vi "Update Servo Parameters.vi"(8 "error in":errorcluster, 11 "tCRD in":refnum<class "Aircraft OPCCRD.lvclass">) -> (0 "error out":errorcluster, 3 "tCRD out":refnum<class "Aircraft OPCCRD.lvclass">)   [LabVIEW 2015, in "Aircraft OPCCRD.lvclass"]
uses:
  Aircraft OPCCRD.lvclass
  Switch/Servo Switch.lvclass
  Reusable/Switch/Switch.lvclass
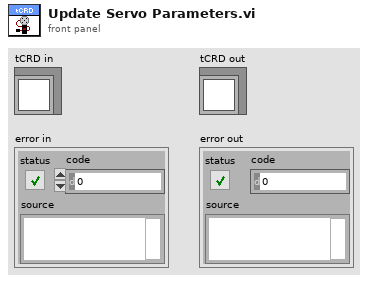
[diagram p1: front panel]
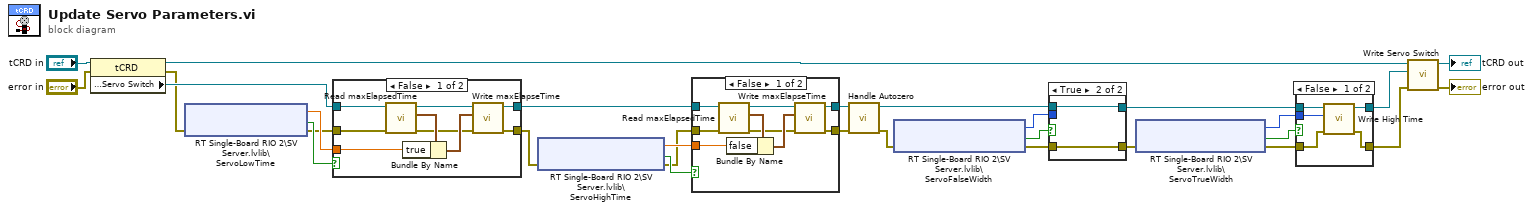
[diagram p0: block diagram]
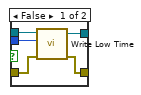
[diagram p3: hidden frame]
diagram:
  n1 = property class="tCRD"(reference="tCRD in", error in="error in") -> (reference out=w4:refnum<class "Aircraft OPCCRD.lvclass">, error out=w1:errorcluster, "Accessors:Servo Switch"=w3:refnum<class "Servo Switch.lvclass">)
  n2 = shared-variable "RT Single-Board RIO 2\\SV Server.lvlib\\ServoLowTime"(error in=w1) -> (w17:sgl, error out=w11:errorcluster, w16:bool)  [unwired: 1 in]
  n3 = case shown="False" w16 {
    tunnel: w11 -> [w34 w40]
    tunnel: [w31 w39] -> w18
    tunnel: w17 -> [w30 _]
    tunnel: w3 -> [w38 w39]
    tunnel: [w32 w40] -> w10
    frame False {
      n4 = call "Read maxElapsedTime.vi"("error in"=w34, "Switch in"=w38) -> ("error out"=w33:errorcluster, "maxElapsedTime"=w37:cluster{"true":sgl, "false":sgl}, "Switch out"=w36:refnum<class "Servo Switch.lvclass">)  [unwired: 7 in]
      n5 = Bundle By Name(cluster=w37, "true"=w30) -> (w35:cluster{"true":sgl, "false":sgl})
      n6 = call "Write maxElapseTime.vi"("error in"=w33, "maxElapsedTime"=w35, "Switch in"=w36) -> ("error out"=w32:errorcluster, "Switch out"=w31:refnum<class "Servo Switch.lvclass">)  [unwired: 7 in]
    }
    frame True {
    }
  }
  n7 = shared-variable "RT Single-Board RIO 2\\SV Server.lvlib\\ServoHighTime"(error in=w10) -> (w19:sgl, error out=w9:errorcluster, w20:bool)  [unwired: 1 in]
  n8 = case shown="False" w20 {
    tunnel: w18 -> [w48 w51]
    tunnel: [w44 w51] -> w21
    tunnel: w19 -> [w49 _]
    tunnel: w9 -> [w47 w50]
    tunnel: [w41 w50] -> w8
    frame False {
      n9 = call "Read maxElapsedTime.vi"("error in"=w47, "Switch in"=w48) -> ("error out"=w42:errorcluster, "maxElapsedTime"=w46:cluster{"true":sgl, "false":sgl}, "Switch out"=w43:refnum<class "Servo Switch.lvclass">)  [unwired: 7 in]
      n10 = Bundle By Name(cluster=w46, "false"=w49) -> (w45:cluster{"true":sgl, "false":sgl})
      n11 = call "Write maxElapseTime.vi"("error in"=w42, "maxElapsedTime"=w45, "Switch in"=w43) -> ("error out"=w41:errorcluster, "Switch out"=w44:refnum<class "Servo Switch.lvclass">)  [unwired: 7 in]
    }
    frame True {
    }
  }
  n12 = call "Handle Autozero.vi"("error in"=w8, "Servo Switch in"=w21) -> ("error out"=w28:errorcluster, "Servo Switch out"=w27:refnum<class "Servo Switch.lvclass">)  [unwired: 8 in]
  n13 = shared-variable "RT Single-Board RIO 2\\SV Server.lvlib\\ServoFalseWidth"(error in=w28) -> (w23:u32, error out=w29:errorcluster, w22:bool)  [unwired: 1 in]
  n14 = case shown="True" w22 {
    tunnel: w27 -> [w56 w58]
    tunnel: w23 -> [w55 _]
    tunnel: [w54 w58] -> w24
    tunnel: w29 -> [w53 w57]
    tunnel: [w52 w57] -> w7
    frame False {
      n15 = call "Write Low Time.vi"("error in (no error)"=w53, "Low Time"=w55, "Servo Switch in"=w56) -> ("error out"=w52:errorcluster, "Servo Switch out"=w54:refnum<class "Servo Switch.lvclass">)  [unwired: 7 in]
    }
    frame True {
    }
  }
  n16 = shared-variable "RT Single-Board RIO 2\\SV Server.lvlib\\ServoTrueWidth"(error in=w7) -> (w26:u32, error out=w6:errorcluster, w25:bool)  [unwired: 1 in]
  n17 = case shown="False" w25 {
    tunnel: w24 -> [w63 w65]
    tunnel: [w62 w65] -> w15
    tunnel: w26 -> [w61 _]
    tunnel: w6 -> [w60 w64]
    tunnel: [w59 w64] -> w14
    frame False {
      n18 = call "Write High Time.vi"("error in (no error)"=w60, "High Time"=w61, "Servo Switch in"=w63) -> ("error out"=w59:errorcluster, "Servo Switch out"=w62:refnum<class "Servo Switch.lvclass">)  [unwired: 7 in]
    }
    frame True {
    }
  }
  n19 = call "Write Servo Switch.vi"("error in (no error)"=w14, "Servo Switch"=w15, "tCRD in"=w4) -> ("error out"=→"error out":errorcluster, "tCRD out"=→"tCRD out":refnum<class "Aircraft OPCCRD.lvclass">)  [unwired: 7 in]
